vi "Normalize Spectrum.vi"(8 "error in (no error)":errorcluster, 10 "Spectrum":dbl[](array[numeric]), 11 "Pressure Gage in":refnum<class "Pressure Gage.lvclass">) -> (0 "error out":errorcluster, 2 "Spectrum out":dbl[](array[numeric]), 3 "Pressure Gage out":refnum<class "Pressure Gage.lvclass">)   [LabVIEW 2016, in "Pressure Gage.lvclass"]
uses:
  Pressure Gage.lvclass
  Pressure Gage.lvclass/Pressure Gage.ctl
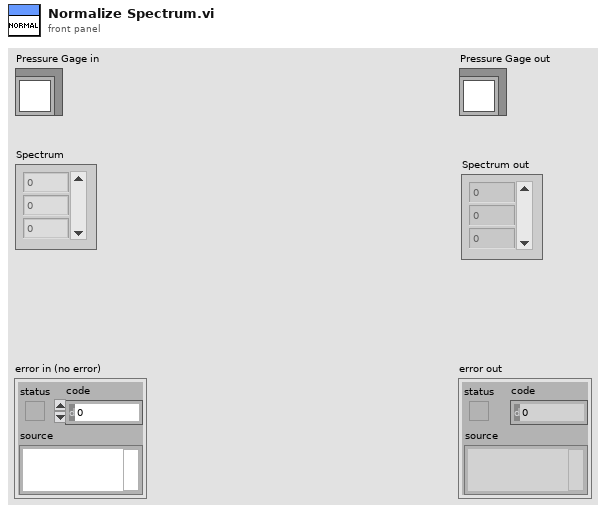
[diagram p1: front panel]
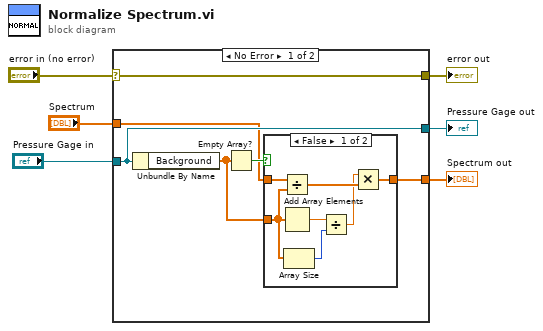
[diagram p0: block diagram]
diagram:
  n1 = case shown="No Error" "error in (no error)" {
    selector: "error in (no error)" -> [w12 w23]
    tunnel: [w12 w23] -> w5
    tunnel: [w11 w22] -> w3
    tunnel: "Pressure Gage in" -> [w11 w22]
    tunnel: "Spectrum" -> [w9 w21]
    tunnel: [w8 w21] -> w1
    frame No Error {
      n2 = Unbundle By Name(w11) -> ("Background"=w7:dbl[])
      n3 = Empty Array?(array=w7) -> (empty?=w10:bool)
      n4 = case shown="False" w10 {
        tunnel: w9 -> [w16 w20]
        tunnel: [w13 w20] -> w8
        tunnel: w7 -> [w17 _]
        frame False {
          n5 = Divide(x=w16, y=w17) -> (x/y=w15:dbl[])
          n6 = Add Array Elements(numeric array=w17) -> (sum=w19:dbl)
          n7 = Array Size(array=w17) -> (size(s)=w18:i32)
          n8 = Divide(x=w19, y=w18) -> (x/y=w14:dbl)
          n9 = Multiply(x=w14, y=w15) -> (x*y=w13:dbl[])
        }
        frame True {
        }
      }
    }
    frame Error {
    }
  }
  "error out" <- w5
  "Pressure Gage out" <- w3
  "Spectrum out" <- w1
